vi "Offset Inline Buffer.vi"(8 "error in (no error)":errorcluster, 9 "group engine offset":u64, 10 "Engine Base Pointer":refnum<class "Pointer.lvclass">, 11 "Transfer in":refnum<class "Transfer.lvclass">) -> (0 "error out":errorcluster, 3 "Transfer out":refnum<class "Transfer.lvclass">)   [LabVIEW 2017, in "DSF Core.lvlib" / "Transfer.lvclass"]
uses:
  Transfer.lvclass
  <vilib>/NI/Memory Manager/Classes/Pointer/Pointer.lvclass
  Transfer.lvclass/Transfer.ctl
  <vilib>/NI/Memory Manager/Classes/Pointer/Pointer.lvclass/Pointer.ctl
  <vilib>/NI/Memory Manager/Classes/Pointer/Get Address.vi
  <vilib>/NI/Memory Manager/Classes/Pointer/Encapsulate.vi
  <vilib>/NI/Memory Manager/Classes/Pointer/Check Null Pointer.vi
  <vilib>/NI/Memory Manager/Classes/Pointer/Check Length.vi
  <vilib>/NI/Memory Manager/Classes/Pointer/Set Size.vi
  <vilib>/NI/Memory Manager/Classes/Pointer/Set Address.vi
  <vilib>/NI/Memory Manager/Classes/Pointer/Set Internal.vi
  <vilib>/NI/Memory Manager/Classes/Pointer/Errors.vi
  <vilib>/NI/Memory Manager/Classes/Pointer/Null Pointer.vi
  <vilib>/NI/Memory Manager/Classes/Pointer/Is Null.vi
  <vilib>/NI/Memory Manager/Classes/Pointer/Check Pointer Bounds.vi
  <vilib>/NI/Memory Manager/Classes/Pointer/Create Error.vi
  <vilib>/NI/Memory Manager/Classes/Pointer/Out of Bounds.vi
  <vilib>/NI/Memory Manager/VIs/New Error Cluster Constant.vi
  <vilib>/NI/Memory Manager/VIs/New Error Cluster Constant (512B).vi
  <vilib>/NI/Memory Manager/VIs/Error Cluster.Set Status.vi
  <vilib>/NI/Memory Manager/VIs/Error Cluster.Set Code.vi
  <vilib>/NI/Memory Manager/VIs/Error Cluster.Set VI Source.vi
  <vilib>/NI/Memory Manager/Constants/Constants.vi
  <vilib>/NI/Memory Manager/Constants/Library Name.vi
  <vilib>/NI/Memory Manager/Classes/Pointer/Pointer Error Info.vi
  <vilib>/NI/Memory Manager/VIs/Source.Write.String.vi
  <vilib>/NI/Memory Manager/Constants/Pointer Class Name.vi
  <vilib>/NI/Memory Manager/Classes/Pointer/Write Pointer Size.vi
  <vilib>/NI/Memory Manager/VIs/Source.Write.Scalar.Base10.vi
  <vilib>/NI/Memory Manager/VIs/Source.Write.Scalar.Base10 (U64).vi
  Pointer/DBL Pointer.lvclass
  C:/Program Files (x86)/National Instruments/LabVIEW 2017/vi.lib/NI/Memory Manager/Classes/Pointer/Pointer.lvclass
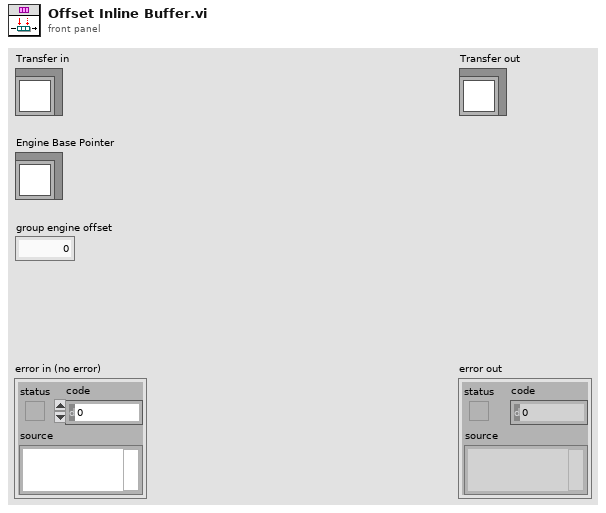
[diagram p1: front panel]
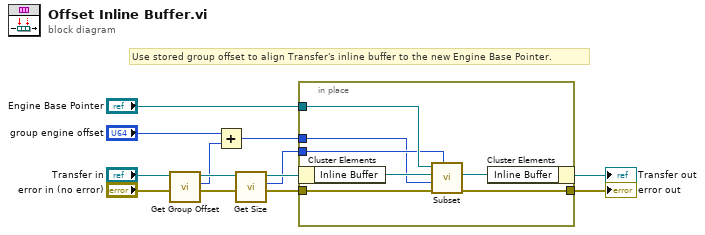
[diagram p0: block diagram]
diagram:
  # "Use stored group offset to align Transfer's inline buffer to the new Engine Base Pointer."
  n1 = call "Get Group Offset.vi"("Transfer in"="Transfer in") -> ("group offset"=w1:u64, "Transfer out"=w7:refnum<class "Transfer.lvclass">)  [unwired: 9 in]
  n2 = Add(x="group engine offset", y=w1) -> (x+y=w5:u64)
  n3 = call <vilib>:"Get Size.vi"("Transfer in"=w7) -> ("size"=w2:u64, "Transfer out"=w4:refnum<class "Transfer.lvclass">)  [unwired: 9 in]
  n4 = in-place {
    in-place-border: "error in (no error)" -> [w18]
    in-place-border: [w17] -> w10
    in-place-border: "Engine Base Pointer" -> [w14]
    in-place-border: w2 -> [w13]
    in-place-border: w5 -> [w12]
    n5 = in-place-cluster #1(w4) -> ("Inline Buffer"=w16:refnum<class "DBL Pointer.lvclass">)
    n6 = call <vilib>:"Subset.vi"("length (-1: rest)"=w13, "error in (no error)"=w18, "offset (0)"=w12, "subset Pointer type"=w16, "base Pointer in"=w14) -> ("error out"=w17:errorcluster, "subset Pointer"=w15:refnum<class "DBL Pointer.lvclass">)  [unwired: 3 in, 2 out]
    n7 = in-place-cluster #1("Inline Buffer"=w15) -> (→"Transfer out":refnum<class "Transfer.lvclass">)
  }
  "error out" <- w10
